vi "Read Frame History Depth.vi"(8 "error in (no error)":errorcluster, 11 "Video Processor in":refnum<class "Video Processor.lvclass">) -> (0 "error out":errorcluster, 2 "Frame History Depth":i32, 3 "Video Processor out":refnum<class "Video Processor.lvclass">)   [LabVIEW 2018, in "Video Processor.lvclass"]
uses:
  Video Processor.lvclass
  Video Processor.lvclass/Video Processor.ctl
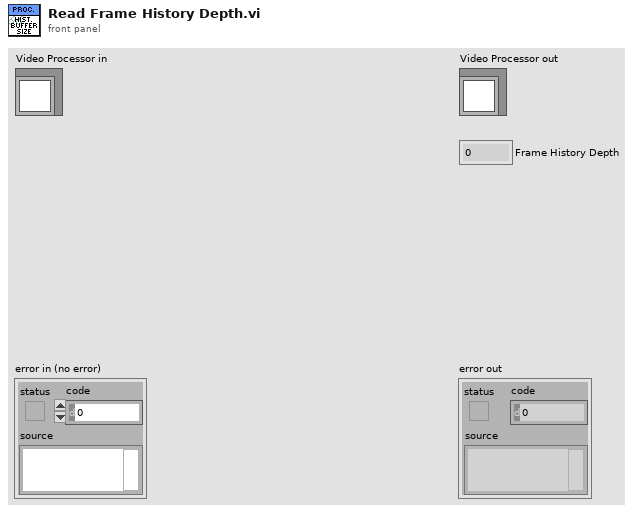
[diagram p1: front panel]
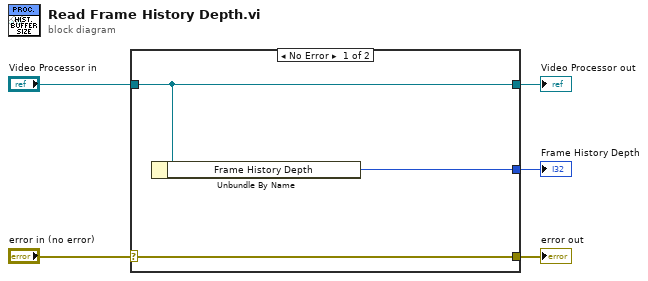
[diagram p0: block diagram]
diagram:
  n1 = case shown="No Error" "error in (no error)" {
    selector: "error in (no error)" -> [w8 w9]
    tunnel: [w8 w9] -> w4
    tunnel: [w7 w10] -> w2
    tunnel: "Video Processor in" -> [w7 w10]
    tunnel: [w6 _] -> w1
    frame No Error {
      n2 = Unbundle By Name(w7) -> ("Frame History Depth"=w6:i32)
    }
    frame Error {
    }
  }
  "error out" <- w4
  "Video Processor out" <- w2
  "Frame History Depth" <- w1
